vi "RemoveFromPalette.vi"(0 "palette path":path, 2 "SubmenuPath":path, 5 "error in (no error)":errorcluster) -> (19 "error out":errorcluster)   [LabVIEW 2012, in "G#Installer.lvlib"]
uses:
  G#Installer.lvlib
  <vilib>/Palette API/Palette Menu/Public Type Define/Palette type.ctl
  <vilib>/Palette API/Palette Menu/Palette Menu.lvlib
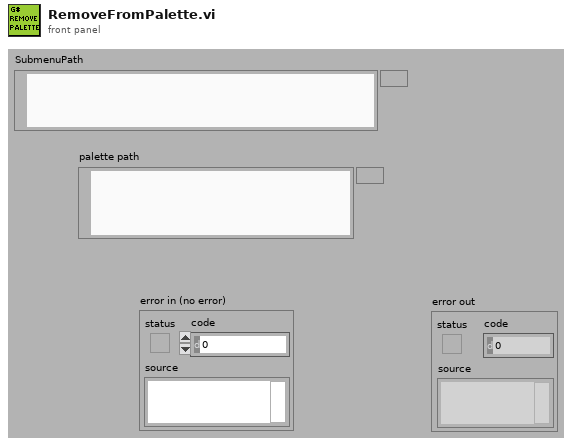
[diagram p1: front panel]
types:
  T1 = typedef "Palette Menu.lvlib/Palette type.ctl" = i32
  T2 = typedef "Palette Menu.lvlib/Palette Data.ctl" = cluster{"display name":string, "view format":T3, "palette width":i16, "items":T4, "256 color icon":picture, "B&W color icon":picture, "help information":T6, "palette description":string, "synchronize information":T7}
  T3 = typedef "Palette Menu.lvlib/View Format.ctl" = u16
  T4 = typedef "Palette Menu.lvlib/Items.ctl" = T5[]
  T5 = typedef "Palette Menu.lvlib/Item.ctl" = cluster{"item path":path, "library path (.lvlib)":path, "use default lvlib palette":bool, "short name":string, "place VI contents":bool, "hide synchronized item":bool, "reserve spot for synch item":bool, "configure when placing VI contents":bool}
  T6 = typedef "Palette Menu.lvlib/Help Info.ctl" = cluster{"help tag":string, "help file path ":path}
  T7 = typedef "Palette Menu.lvlib/Synchronize Info.ctl" = cluster{"synchronize with directory":bool, "synchronize directory path":path}
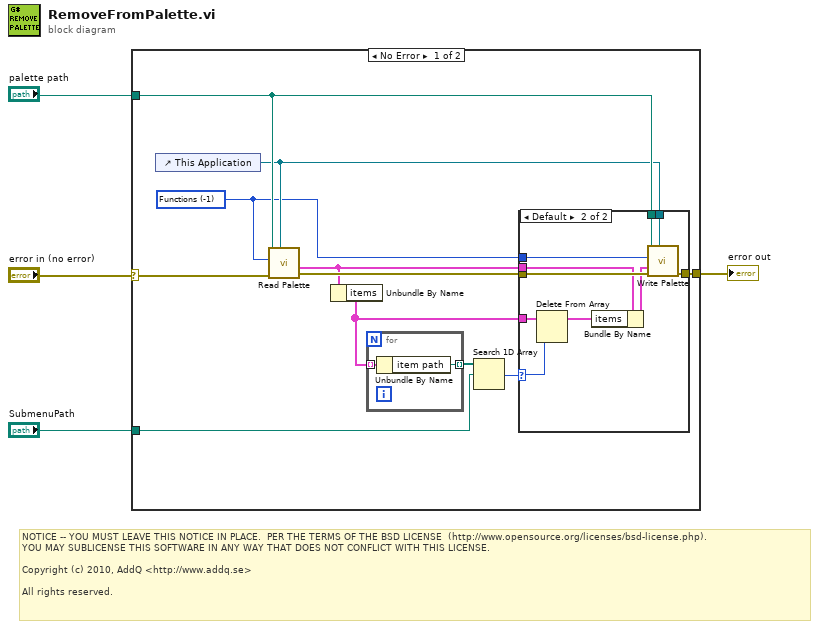
[diagram p0: block diagram]
diagram:
  # "NOTICE -- YOU MUST LEAVE THIS NOTICE IN PLACE.  PER THE TERMS OF THE BSD LICENSE  (http://www.opensource.org/licenses/bsd-license.php).\nYOU MAY SUBLICENSE THIS SOFTWARE IN ANY WAY THAT DOES NOT CONFLICT WITH THIS LICENSE.\n\nCopyright (c) 2010, AddQ <http://www.addq.se>\n\nAll rights reserved."
  n1 = case shown="No Error" "error in (no error)" {
    selector: "error in (no error)" -> [w9 w29]
    tunnel: "SubmenuPath" -> [w7 _]
    tunnel: "palette path" -> [w15 _]
    tunnel: [w10 w29] -> w2
    frame No Error {
      w12 = T1 -1 items=["Functions"=-1, "Controls"=-2] ("palette type")
      n2 = control-ref of="This Application"() -> (w14:refnum<vi>)
      n3 = call <vilib>:"Read Palette.vi"("application reference"=w14, "error in (no error)"=w9, "palette type"=w12, "palette path"=w15) -> ("error out"=w13:errorcluster, "palette data"=w11:T2)  [unwired: 5 in, 1 out]
      n4 = Unbundle By Name(w11) -> ("items"=w6:T4)
      n5 = for {
        tunnel: w6 -> [w28] mode=indexing
        tunnel: [w27] -> w8 mode=indexing
        n6 = Unbundle By Name(w28) -> ("item path"=w27:path)
      }
      n7 = Search 1D Array(1D array=w8, element=w7) -> (index of element=w5:i32)  [unwired: 1 in]
      n8 = case shown="Default" w5 {
        selector: w5 -> [_ w17]
        tunnel: w15 -> [_ w26]
        tunnel: w14 -> [_ w25]
        tunnel: w13 -> [w16 w24]
        tunnel: w12 -> [_ w23]
        tunnel: w11 -> [_ w22]
        tunnel: [w16 w20] -> w10
        tunnel: w6 -> [_ w19]
        frame -1 {
        }
        frame Default {
          n9 = Delete From Array(array=w19, index=w17) -> (array with subset deleted=w18:T4)  [unwired: 1 in, 1 out]
          n10 = Bundle By Name(cluster=w22, "items"=w18) -> (w21:T2)
          n11 = call <vilib>:"Write Palette.vi"("application reference"=w25, "error in (no error)"=w24, "palette data"=w21, "palette type"=w23, "palette path"=w26) -> ("error out"=w20:errorcluster)  [unwired: 6 in]
        }
      }
    }
    frame Error {
    }
  }
  "error out" <- w2
